vi "AVS_PrepareMeasure.vi"(0 "a_hDevice":i32, 7 "a_pMeasConfig":T1) -> (4 "Output Value":i32)   [LabVIEW 2013, in "Avantes Spectrometer Functions.lvlib"]
uses:
  Avantes Spectrometer Functions.lvlib
  AS5216.dll
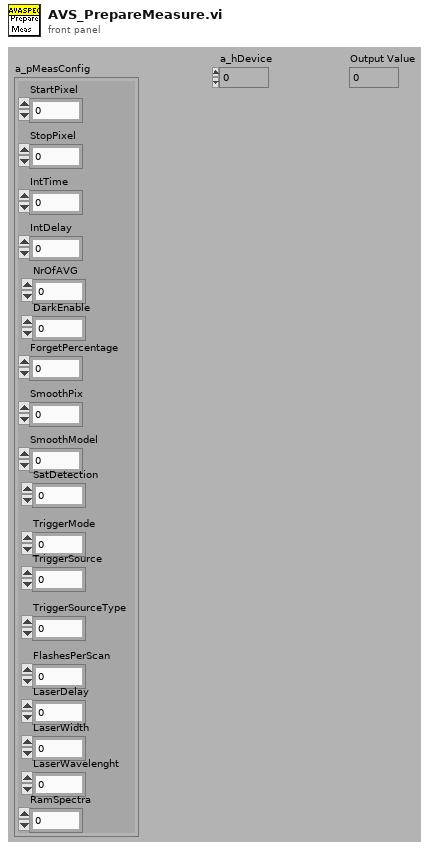
[diagram p1: front panel]
types:
  T1 = cluster{"StartPixel":u16, "StopPixel":u16, "IntTime":sgl, "IntDelay":u32, "NrOfAVG":u32, "DarkEnable":u8, "ForgetPercentage":u8, "SmoothPix":u16, "SmoothModel":u8, "SatDetection":u8, "TriggerMode":u8, "TriggerSource":u8, "TriggerSourceType":u8, "FlashesPerScan":u16, "LaserDelay":u32, "LaserWidth":u32, "LaserWavelenght":sgl, "RamSpectra":u16}
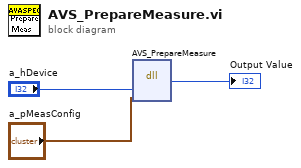
[diagram p0: block diagram]
diagram:
  n1 = dll-call lib="C:/Users/dhstuart/Dropbox/CLTC/avantesSpectrometer/Libraries/AS-5216-DLL/polling_mc/AS5216.dll" fn="AVS_PrepareMeasure"("a_hDevice"="a_hDevice", "a_pMeasConfig"="a_pMeasConfig") -> (→"Output Value":i32)  [unwired: 5 in, 2 out]
